vi "Fill Hole VI.vi"(3 "error in (no error)":errorcluster, 5 "Image In":T1) -> (0 "error out":errorcluster, 2 "Fill holes\nimage":T1(plugin-control))   [LabVIEW 2020]
uses:
  <vilib>/vision/Image Controls.llb/IMAQ Image.ctl
  <vilib>/vision/NI_Vision_Development_Module.lvlib
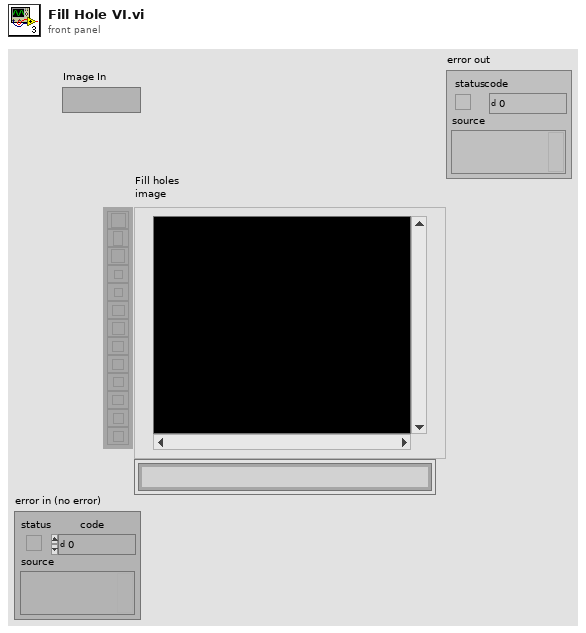
[diagram p1: front panel]
types:
  T1 = typedef "IMAQ Image.ctl" = refnum<image>
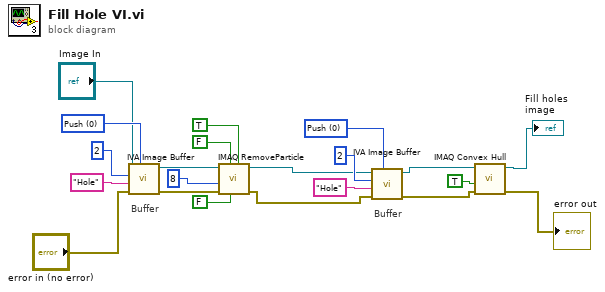
[diagram p0: block diagram]
diagram:
  w7 = u16 0 items=["Push", "Pop", "Reset"] ("Function")
  w16 = u16 0 items=["Push", "Pop", "Reset"] ("Function")
  # "Buffer"
  # "Buffer"
  n1 = call <vilib>:"IVA Image Buffer.vi"("Function"=w16, "error in (no error)"="error in (no error)", "Prefix"="Hole", "Buffer #"=2, "Image In"="Image In") -> ("error out"=w13:errorcluster, "Image Out"=w12:T1)  [unwired: 5 out]
  n2 = call "IMAQ RemoveParticle"("Connectivity 4/8 (8)"=TRUE, "Low Pass/High Pass (Low)"=FALSE, "Square/Hexa (Square)"=FALSE, "error in (no error)"=w13, "Number of Erosion"=8, "Image Src"=w12) -> ("error out"=w4:errorcluster, "Image Dst Out"=w3:T1)  [unwired: 1 in, 3 out]
  n3 = call <vilib>:"IVA Image Buffer.vi"("Function"=w7, "error in (no error)"=w4, "Prefix"="Hole", "Buffer #"=2, "Image In"=w3) -> ("error out"=w1:errorcluster, "Image Out"=w2:T1)  [unwired: 5 out]
  n4 = call "IMAQ Convex Hull"("error in (no error)"=w1, "Connectivity 4/8 (8)"=TRUE, "Image Src"=w2) -> ("error out"=→"error out":errorcluster, "Image Dst Out"=→"Fill holes\nimage":T1)  [unwired: 1 in, 6 out]
